vi "Register Events to Controller.vi"(8 "error in (no error)":errorcluster, 11 "Example View in":refnum<class "Example GUI View.lvclass">) -> (0 "error out":errorcluster, 3 "Example View out":refnum<class "Example GUI View.lvclass">)   [LabVIEW 2023, in "Example GUI View.lvlib" / "Example GUI View.lvclass"]
doc: "This dinamic dispatch methods has to be overriddent by the child sink classes to register events to the source"
uses:
  Example GUI View.lvclass
  Example GUI View Messages/Update Array Event Msg/Update Array Event Msg.lvclass
  Example Events/Double Array Event.lvclass
  Example GUI View Messages/Update Time Event Msg/Update Time Event Msg.lvclass
  Example Events/Timestamp Event.lvclass
  Example GUI View Messages/Update Boolean Event Msg/Update Boolean Event Msg.lvclass
  Example Events/Boolean Event.lvclass
  Event/Event.lvclass/Event.ctl
  Event/Event.lvclass
  View/View.lvclass
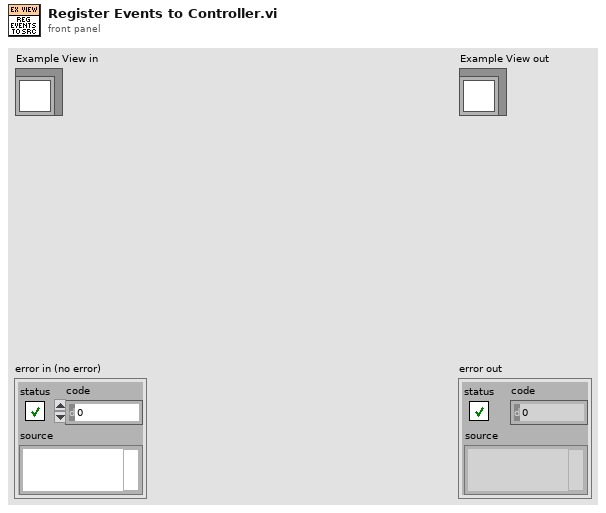
[diagram p1: front panel]
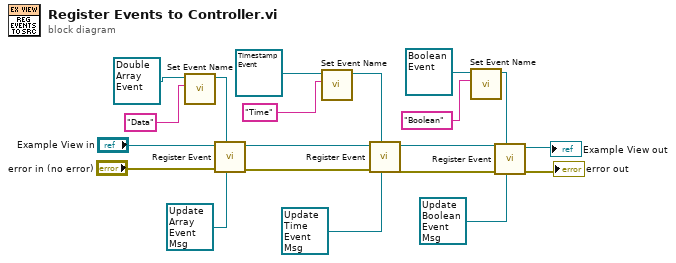
[diagram p0: block diagram]
diagram:
  n1 = call "Set Event Name.vi"("Name (Generic)"="Data", "Event In"=refnum<class "Double Array Event.lvclass"> refnum ("Double Array Event.lvclass")) -> ("Event Out"=w16:refnum<class "Double Array Event.lvclass">)  [unwired: 9 in]
  n2 = call "Register Event.vi"("Event Handler"=refnum<class "Update Array Event Msg.lvclass"> refnum ("Update Array Msg.lvclass"), "Event"=w16, "error in (no error)"="error in (no error)", "View in"="Example View in") -> ("error out"=w13:errorcluster, "View out"=w14:refnum<class "Example GUI View.lvclass">)  [unwired: 6 in]
  n3 = call "Set Event Name.vi"("Name (Generic)"="Time", "Event In"=refnum<class "Timestamp Event.lvclass"> refnum ("Timestamp Event.lvclass")) -> ("Event Out"=w10:refnum<class "Timestamp Event.lvclass">)  [unwired: 9 in]
  n4 = call "Register Event.vi"("Event Handler"=refnum<class "Update Time Event Msg.lvclass"> refnum ("Update Time Msg.lvclass"), "Event"=w10, "error in (no error)"=w13, "View in"=w14) -> ("error out"=w5:errorcluster, "View out"=w6:refnum<class "Example GUI View.lvclass">)  [unwired: 6 in]
  n5 = call "Set Event Name.vi"("Name (Generic)"="Boolean", "Event In"=refnum<class "Boolean Event.lvclass"> refnum ("Example Source.lvlib:Boolean Event.lvclass")) -> ("Event Out"=w4:refnum<class "Boolean Event.lvclass">)  [unwired: 9 in]
  n6 = call "Register Event.vi"("Event Handler"=refnum<class "Update Boolean Event Msg.lvclass"> refnum ("Update Time Msg.lvclass"), "Event"=w4, "error in (no error)"=w5, "View in"=w6) -> ("error out"=→"error out":errorcluster, "View out"=→"Example View out":refnum<class "Example GUI View.lvclass">)  [unwired: 6 in]
